vi "Auto Shoot.vi"() -> (2 "Left Speed":dbl, 3 "Right Speed":dbl)   [LabVIEW 2016]
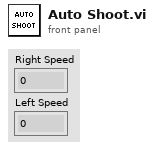
[diagram p1: front panel]
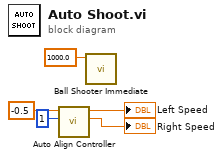
[diagram p0: block diagram]
diagram:
  n1 = call "Auto Align Controller.vi"("Step (in)"=1, "Base Speed"=-0.5) -> ("Right Speed"=→"Right Speed":dbl, "Left Speed"=→"Left Speed":dbl)  [unwired: 7 in, 1 out]
  n2 = call "Ball Shooter Immediate.vi"("Duration"=1000.0) -> ()  [unwired: 10 in, 1 out]
